vi "Stop Motion.vi"(8 "error in (no error)":errorcluster, 11 "VISA resource name":refnum<visa-resource-name>) -> (0 "error out":errorcluster, 3 "VISA resource out":refnum<visa-resource-name>)   [LabVIEW 2017]
doc: "Interrupt current motion.\nQuit onl-line mode and return to Local mode.\nClose VISA session."
panel:
  out "Response String ('/' codes)":string
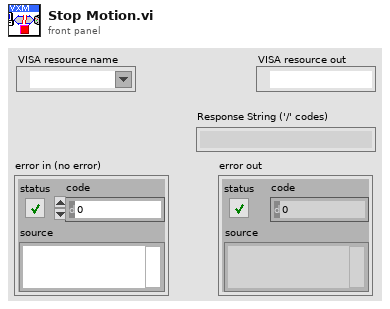
[diagram p1: front panel]
types:
  T1 = enum16{"Cmd-Response", "Write Only", "Read Only"}
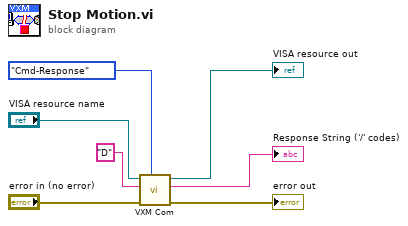
[diagram p0: block diagram]
diagram:
  n1 = call "VXM Com.vi"("Operation"=T1."Cmd-Response", "error in (no error)"="error in (no error)", "Write Buffer ('/' codes)"="D" ("Write Buffer"), "VISA resource name"="VISA resource name") -> ("error out"=→"error out":errorcluster, "Response String ('/' codes)"=→"Response String ('/' codes)":string, "VISA resource out"=→"VISA resource out":refnum<visa-resource-name>)  [unwired: 5 in]
